vi "tabcontrol.vi"() -> ()   [LabVIEW 2017]
panel:
  out "String":string
  in  "stop":bool
  in  "C mamo":enum32{"Radiohead", "Judas Priest", "Tool"}(tab)
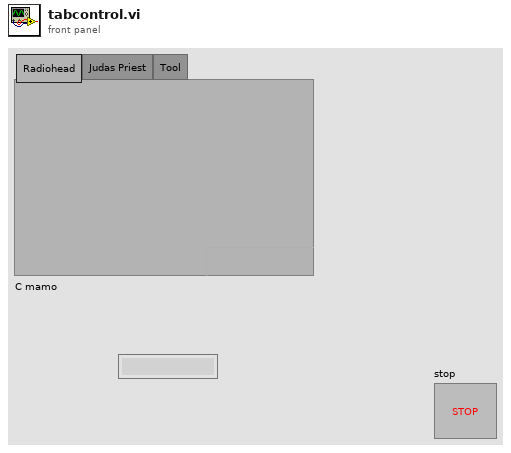
[diagram p1: front panel]
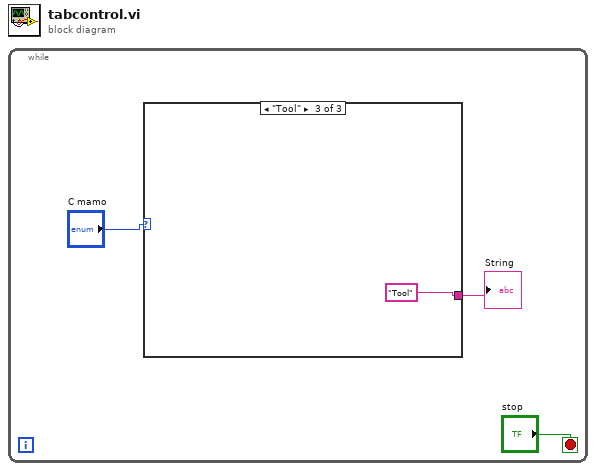
[diagram p0: block diagram]
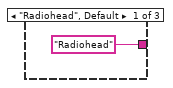
[diagram p2: hidden frame]
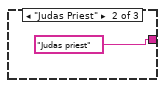
[diagram p3: hidden frame]
diagram:
  n1 = while {
    stop <- "stop" stop-if-true
    n2 = case shown="\"Tool\"" "C mamo" {
      tunnel: ["Radiohead" "Judas priest" "Tool"] -> w1
      frame "Radiohead", Default {
      }
      frame "Judas Priest" {
      }
      frame "Tool" {
      }
    }
    "String" <- w1
  }
